vi "Find ADC Code Transition.vi"(9 "ADC data":T1[](array[typedef]), 11 "code before transition":u32) -> (3 "transition voltage":dbl format="%.9f")   [LabVIEW 2021, in "adc_fullScaleError.lvlib"]
uses:
  adc_fullScaleError.lvlib
  Controls/ADC Data.ctl
  0dce6366-741c-4d91-83ba-59aba7831395.vi
  ee4e2351-e801-4e3f-a4e3-5e4118ca8a7c.vi
  db61ecb9-b899-4ec6-b81d-f6250db39a66.vi
  <vilib>/Comparison/Less/Less Functor/Less Functor.lvclass
  <vilib>/Analysis/baseanly.llb/Mean (DBL).vi
  <vilib>/Analysis/NI_AALBase.lvlib
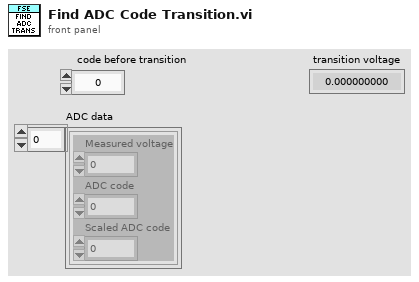
[diagram p1: front panel]
types:
  T1 = typedef "adc_fullScaleError.lvlib/ADC Data.ctl" = cluster{"Measured voltage":dbl, "ADC code":u32, "Scaled ADC code":dbl}
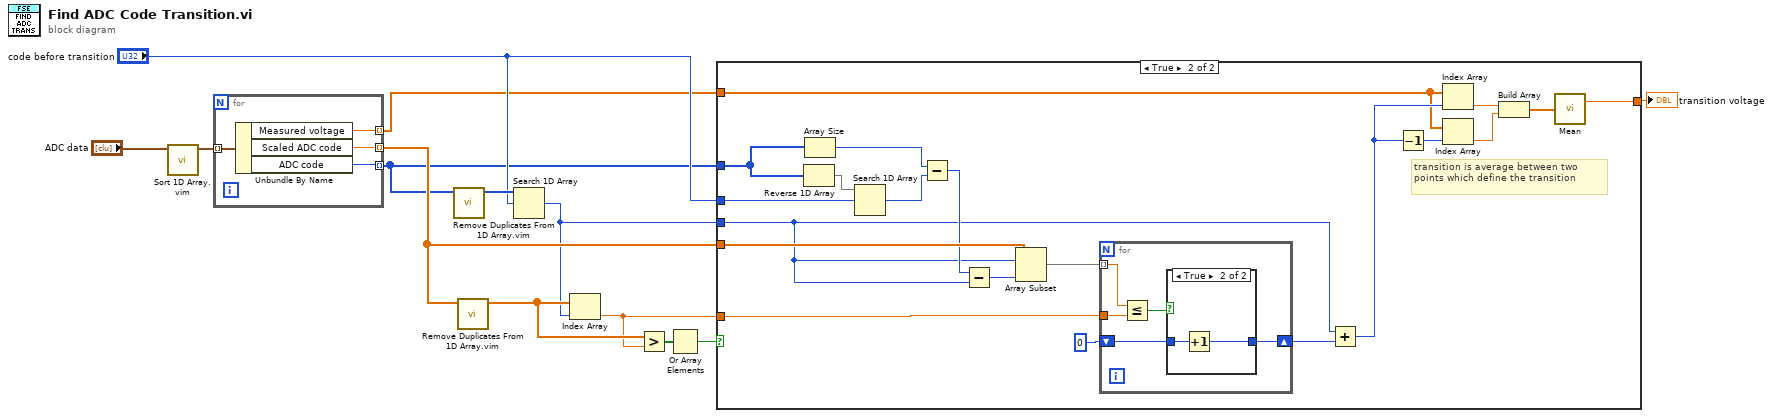
[diagram p0: block diagram]
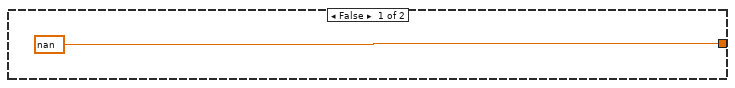
[diagram p2: hidden frame]
diagram:
  n1 = call "Sort 1D Array.vim"("unsorted array"="ADC data") -> ("sorted array"=w5:T1[])  [unwired: 10 in]
  n2 = for {
    tunnel: w5 -> [w17] mode=indexing
    tunnel: [w16] -> w4 mode=indexing
    tunnel: [w15] -> w3 mode=indexing
    tunnel: [w14] -> w2 mode=indexing
    n3 = Unbundle By Name(w17) -> ("Measured voltage"=w16:dbl, "Scaled ADC code"=w15:dbl, "ADC code"=w14:u32)
  }
  n4 = call "Remove Duplicates From 1D Array.vim"("array"=w2) -> ("array with duplicates removed"=w12:u32[])  [unwired: 10 in]
  n5 = call "Remove Duplicates From 1D Array.vim"("array"=w3) -> ("array with duplicates removed"=w11:dbl[])  [unwired: 10 in]
  n6 = Search 1D Array(1D array=w12, element="code before transition") -> (index of element=w1:i32)  [unwired: 1 in]
  n7 = Index Array(array=w11, index=w1) -> (element=w7:dbl)
  n8 = Greater?(x=w11, y=w7) -> (0:w10:bool[])
  n9 = Or Array Elements(Boolean array=w10) -> (logical OR=w9:bool)
  n10 = case shown="True" w9 {
    tunnel: w4 -> [_ w35]
    tunnel: [nan ("mean") w32] -> w13
    tunnel: w2 -> [_ w29]
    tunnel: "code before transition" -> [_ w27]
    tunnel: w3 -> [_ w26]
    tunnel: w7 -> [_ w23]
    tunnel: w1 -> [_ w19]
    frame False {
    }
    frame True {
      # "transition is average between two points which define the transition"
      n11 = Reverse 1D Array(array=w29) -> (reversed array=w28:u32[])
      n12 = Array Size(array=w29) -> (size(s)=w30:i32)
      n13 = Search 1D Array(1D array=w28, element=w27) -> (index of element=w31:i32)  [unwired: 1 in]
      n14 = Subtract(x=w30, y=w31) -> (x-y=w20:i32)
      n15 = Subtract(x=w20, y=w19) -> (x-y=w25:i32)
      n16 = Array Subset(array=w26, index=w19, length=w25) -> (w24:dbl[])
      n17 = for {
        tunnel: w24 -> [w43] mode=indexing
        tunnel: w23 -> [w42]
        shift-right: [w39] -> w21
        shift-left: 0 -> [w40]
        n18 = Less Or Equal?(x=w43, y=w42) -> (x <= y?=w41:bool)
        n19 = case shown="True" w41 {
          tunnel: w40 -> [w44 w46]
          tunnel: [w44 w45] -> w39
          frame False {
          }
          frame True {
            n20 = Increment(x=w46) -> (x+1=w45:i32)
          }
        }
      }
      n21 = Add(x=w19, y=w21) -> (x+y=w37:i32)
      n22 = Decrement(x=w37) -> (x-1=w38:i32)
      n23 = Index Array(array=w35, index=w37) -> (element=w36:dbl)
      n24 = Index Array(array=w35, index=w38) -> (element=w34:dbl)
      n25 = Build Array(w36, w34) -> (w33:dbl[])
      n26 = call-poly <vilib>:"Mean.vi"("X"=w33) -> ("mean"=w32:dbl)  [unwired: 1 out]
    }
  }
  "transition voltage" <- w13
